vi "SetAttributeViReal64_SE_SpE_Trigger_OB.vi"(7 "AttributeValue":dbl, 8 "error in (no error)":errorcluster {"code" format="%.0x"}, 9 "AttributeID":u32(ring)=1190391 items=["OCCUPIED_BANDWIDTH_DISPLAY_WINDOWY_REFERENCE"=1190391, "OCCUPIED_BANDWIDTH_DISPLAY_WINDOWY_SCALE"=1190392, "OCCUPIED_BANDWIDTH_FREQUENCY_SPAN"=1190394, "OCCUPIED_BANDWIDTH_FREQUENCY_XDB"=1190387, "OCCUPIED_BANDWIDTH_LIMIT_TEST_FREQUENCY"=1190384, "OCCUPIED_BANDWIDTH_MARKER_POSITION"=1190400, "OCCUPIED_BANDWIDTH_MARKER_TRACE_POINTS_POSITION"=1190663, "OCCUPIED_BANDWIDTH_PERCENT_POWER"=1190386, "OCCUPIED_BANDWIDTH_SWEEPCOUPLING_RESOLUTION_BANDWIDTH"=1190409, "OCCUPIED_BANDWIDTH_SWEEPCOUPLING_SWEEP_TIME"=1190412, "OCCUPIED_BANDWIDTH_SWEEPCOUPLING_VIDEO_BANDWIDTH"=1190414, "SEMASK_DISPLAY_WINDOWX_REFERENCE"=1191466, "SEMASK_DISPLAY_WINDOWX_SCALE"=1191468, "SEMASK_DISPLAY_WINDOWY_REFERENCE"=1190487, "SEMASK_DISPLAY_WINDOWY_SCALE"=1190488, "SEMASK_MARKER_POSITION"=1190497, "SEMASK_MARKER_TRACE_POINTS_POSITION"=1191510, "SEMASK_OFFSET_FILTER_ALPHA"=1190498, "SEMASK_REFERENCE_CHANNEL_CPSD"=1190478, "SEMASK_REFERENCE_CHANNEL_FREQUENCY_SPAN"=1150032, "SEMASK_REFERENCE_CHANNEL_PEAK_POWER"=1150122, "SEMASK_REFERENCE_CHANNEL_TOTAL_POWER"=1190481, "SEMASK_SWEEPCOUPLING_BANDWIDTH_RATIO"=1150118, "SEMASK_SWEEPCOUPLING_CHANNEL_INTEGRATION_BANDWIDTH"=1190486, "SEMASK_SWEEPCOUPLING_RESOLUTION_BANDWIDTH"=1190479, "SEMASK_SWEEPCOUPLING_SWEEP_TIME"=1190483, "SEMASK_SWEEPCOUPLING_VIDEO_BANDWIDTH"=1150120, "SPURIOUS_EMISSIONS_DISPLAY_WINDOWY_REFERENCE"=1190520, "SPURIOUS_EMISSIONS_DISPLAY_WINDOWY_SCALE"=1190521, "SPURIOUS_EMISSIONS_MARKER_POSITION"=1190530, "SPURIOUS_EMISSIONS_MARKER_TRACE_POINTS_POSITION"=1190667, "TRIGGER_AIQ_MAGNITUDE_BANDWIDTH"=1190814, "TRIGGER_AIQ_MAGNITUDE_CENTER_FREQUENCY"=1190815, "TRIGGER_AIQ_MAGNITUDE_DELAY"=1190816, "TRIGGER_AIQ_MAGNITUDE_LEVEL"=1190818, "TRIGGER_AUTO_TIME"=1190137, "TRIGGER_EXTERNAL2_DELAY"=1190142, "TRIGGER_EXTERNAL2_LEVEL"=1190144, "TRIGGER_EXTERNAL_DELAY"=1190138, "TRIGGER_EXTERNAL_LEVEL"=1190140, "TRIGGER_FRAME_DELAY"=1190146, "TRIGGER_FRAME_OFFSET"=1190580, "TRIGGER_FRAME_PERIOD"=1190148, "TRIGGER_FRAME_RFBURST_LEVEL_ABSOLUTE"=1191763, "TRIGGER_FRAME_SYNCHOLDOFF_TIME"=1190611, "TRIGGER_HOLDOFF_TIME"=1190157, "TRIGGER_I_DEMODULATED_DELAY"=1190822, "TRIGGER_I_DEMODULATED_LEVEL"=1190820, "TRIGGER_INPUT_I_DELAY"=1190824, "TRIGGER_INPUT_I_LEVEL"=1190826, "TRIGGER_INPUT_Q_DELAY"=1190836, "TRIGGER_INPUT_Q_LEVEL"=1190838, "TRIGGER_IQ_MAGNITUDE_DELAY"=1190828, "TRIGGER_IQ_MAGNITUDE_LEVEL"=1190830, "TRIGGER_LINE_DELAY"=1190158, "TRIGGER_Q_DEMODULATED_DELAY"=1190832, "TRIGGER_Q_DEMODULATED_LEVEL"=1190834, "TRIGGER_RFBURST_DELAY"=1190161, "TRIGGER_RFBURST_LEVEL_ABSOLUTE"=1190164, "TRIGGER_RFBURST_LEVEL_RELATIVE"=1190165, "TRIGGER_VIDEO_DELAY"=1190167, "TRIGGER_VIDEO_LEVEL"=1190169], 10 "RepCapIdentifier":string, 11 "instrument handle":refnum<k15>) -> (0 "error out":errorcluster {"code" format="%.0x"}, 3 "instrument handle out":refnum<k15>)   [LabVIEW 2021, in "Keysight XSAnVMA.lvlib"]
doc: "Sets Real64 Attribute from instrumrnt driver.\nThe following attributes are supported:\n\nOCCUPIED_BANDWIDTH_DISPLAY_WINDOWY_REFERENCE\nOCCUPIED_BANDWIDTH_DISPLAY_WINDOWY_SCALE\nOCCUPIED_BANDWIDTH_FREQUENCY_SPAN\nOCCUPIED_BANDWIDTH_FREQUENCY_XDB\nOCCUPIED_BANDWIDTH_LIMIT_TEST_FREQUENCY\nOCCUPIED_BANDWIDTH_MARKER_POSITION\nOCCUPIED_BANDWIDTH_MARKER_TRACE_POINTS_POSITION\nOCCUPIED_BANDWIDTH_PERCENT_POWER\nOCCUPIED_BANDWIDTH_SWEEPCOUPLING_RESOLUTION_BANDWIDTH\nOCCUPIED_BANDWIDTH_SWEEPCOUPLING_SWEEP_TIME\nOCCUPIED_BANDWIDTH_SWEEPCOUPLING_VIDEO_BANDWIDTH\nSEMASK_DISPLAY_WINDOWX_REFERENCE\nSEMASK_DISPLAY_WINDOWX_SCALE\nSEMASK_DISPLAY_WINDOWY_REFERENCE\nSEMASK_DISPLAY_WINDOWY_SCALE\nSEMASK_MARKER_POSITION\nSEMASK_MARKER_TRACE_POINTS_POSITION\nSEMASK_OFFSET_FILTER_ALPHA\nSEMASK_REFERENCE_CHANNEL_CPSD\nSEMASK_REFERENCE_CHANNEL_FREQUENCY_SPAN\nSEMASK_REFERENCE_CHANNEL_PEAK_POWER\nSEMASK_REFERENCE_CHANNEL_TOTAL_POWER\nSEMASK_SWEEPCOUPLING_BANDWIDTH_RATIO\nSEMASK_SWEEPCOUPLING_CHANNEL_INTEGRATION_BANDWIDTH\nSEMASK_SWEEPCOUPLING_RESOLUTION_BANDWIDTH\nSEMASK_SWEEPCOUPLING_SWEEP_TIME\nSEMASK_SWEEPCOUPLING_VIDEO_BANDWIDTH\nSPURIOUS_EMISSIONS_DISPLAY_WINDOWY_REFERENCE\nSPURIOUS_EMISSIONS_DISPLAY_WINDOWY_SCALE\nSPURIOUS_EMISSIONS_MARKER_POSITION\nSPURIOUS_EMISSIONS_MARKER_TRACE_POINTS_POSITION\nTRIGGER_AIQ_MAGNITUDE_BANDWIDTH\nTRIGGER_AIQ_MAGNITUDE_CENTER_FREQUENCY\nTRIGGER_AIQ_MAGNITUDE_DELAY\nTRIGGER_AIQ_MAGNITUDE_LEVEL\nTRIGGER_AUTO_TIME\nTRIGGER_EXTERNAL2_DELAY\nTRIGGER_EXTERNAL2_LEVEL\nTRIGGER_EXTERNAL_DELAY\nTRIGGER_EXTERNAL_LEVEL\nTRIGGER_FRAME_DELAY\nTRIGGER_FRAME_OFFSET\nTRIGGER_FRAME_PERIOD\nTRIGGER_FRAME_RFBURST_LEVEL_ABSOLUTE\nTRIGGER_FRAME_SYNCHOLDOFF_TIME\nTRIGGER_HOLDOFF_TIME\nTRIGGER_I_DEMODULATED_DELAY\nTRIGGER_I_DEMODULATED_LEVEL\nTRIGGER_INPUT_I_DELAY\nTRIGGER_INPUT_I_LEVEL\nTRIGGER_INPUT_Q_DELAY\nTRIGGER_INPUT_Q_LEVEL\nTRIGGER_IQ_MAGNITUDE_DELAY\nTRIGGER_IQ_MAGNITUDE_LEVEL\nTRIGGER_LINE_DELAY\nTRIGGER_Q_DEMODULATED_DELAY\nTRIGGER_Q_DEMODULATED_LEVEL\nTRIGGER_RFBURST_DELAY\nTRIGGER_RFBURST_LEVEL_ABSOLUTE\nTRIGGER_RFBURST_LEVEL_RELATIVE\nTRIGGER_VIDEO_DELAY\nTRIGGER_VIDEO_LEVEL"
uses:
  <instrlib>/Keysight XSAnVMA/Keysight XSAnVMA.lvlib
  KtXSAnVMA_64.dll
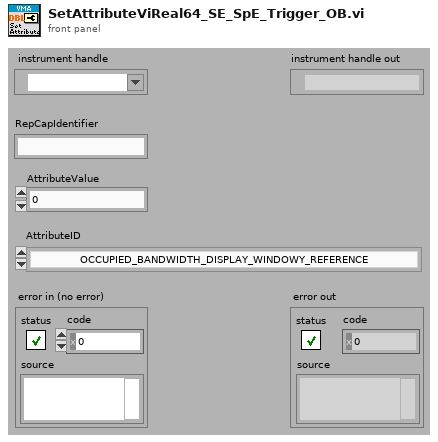
[diagram p1: front panel]
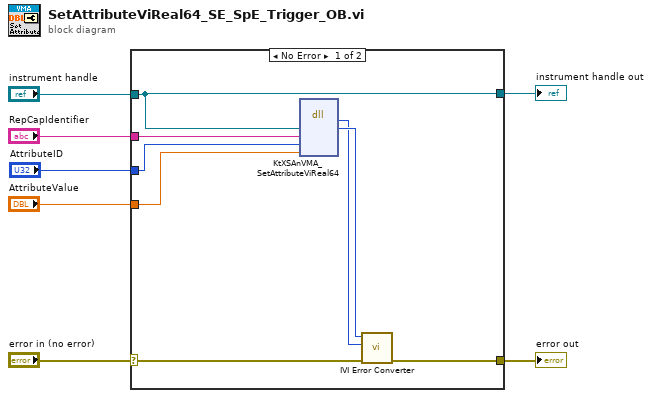
[diagram p0: block diagram]
diagram:
  n1 = case shown="No Error" "error in (no error)" {
    selector: "error in (no error)" -> [w13 w17]
    tunnel: [w12 w17] -> w7
    tunnel: "instrument handle" -> [w8 w16]
    tunnel: "RepCapIdentifier" -> [w11 _]
    tunnel: "AttributeID" -> [w10 _]
    tunnel: "AttributeValue" -> [w9 _]
    tunnel: [w8 w16] -> w2
    frame No Error {
      n2 = dll-call lib="KtXSAnVMA**.dll" fn="KtXSAnVMA_SetAttributeViReal64"("Vi"=w8, "RepCapIdentifier"=w11, "AttributeID"=w10, "AttributeValue"=w9) -> ("return type"=w14:i32, "Vi"=w15:u32)  [unwired: 6 in, 2 out]
      n3 = call <instrlib>:"IVI Error Converter.vi"("error in (no error)"=w13, "IVI error code (0)"=w14, "instrument handle"=w15) -> ("error out"=w12:errorcluster)  [unwired: 7 in, 1 out]
    }
    frame Error {
    }
  }
  "error out" <- w7
  "instrument handle out" <- w2
